vi "FUG-HCN.ProcCases.vi"(0 "i ref in":refnum<vi>, 1 "selector":string, 2 "Data":T1, 3 "call cluster":T2={"Object"="", "Selector"="", "CallType"=enum."synchronous", "Async Object"="", "Async Selector"="", "Data Descriptor"="", "Data"=[], "Error #"=0, "Expire"=0}, 5 "error in (no error)":errorcluster) -> (14 "i ref out":refnum<vi>, 17 "answer cluster":T2={"Object"="", "Selector"="", "CallType"=enum."synchronous", "Async Object"="", "Async Selector"="", "Data Descriptor"="", "Data"=[], "Error #"=0, "Expire"=0}, 19 "error out":errorcluster)   [LabVIEW 2014, in "FUG-HCN.lvlib"]
doc: "This method is called by a process from within the default case in the event loop. The methods of a class that are linked to events will be called from THIS method. Add your code here."
uses:
  FUG-HCN.lvlib
  CS_Core/BaseProcess/BaseProcess.lvlib
  CS_Core/CSSystem/CoreLib/CoreLib.lvlib
  CS_Core/CSSystem/CoreLib/CoreLib.string 2 byte array.vi
  CS_Core/CSSystem/CoreLib/CoreLib.double 2 byte array.vi
  CS_Core/CSSystem/CoreLib/CoreLib.byte array 2 short.vi
  CS_Core/CSSystem/CoreLib/CoreLib.byte array 2 double.vi
  CS_Core/CSSystem/CoreDefs/CoreDefs.call_type.ctl
  CS_Core/BaseProcess/BaseProcess.descriptor string definition.ctl
  CS_Core/CSSystem/CoreDefs/CoreDefs.rawDataType.ctl
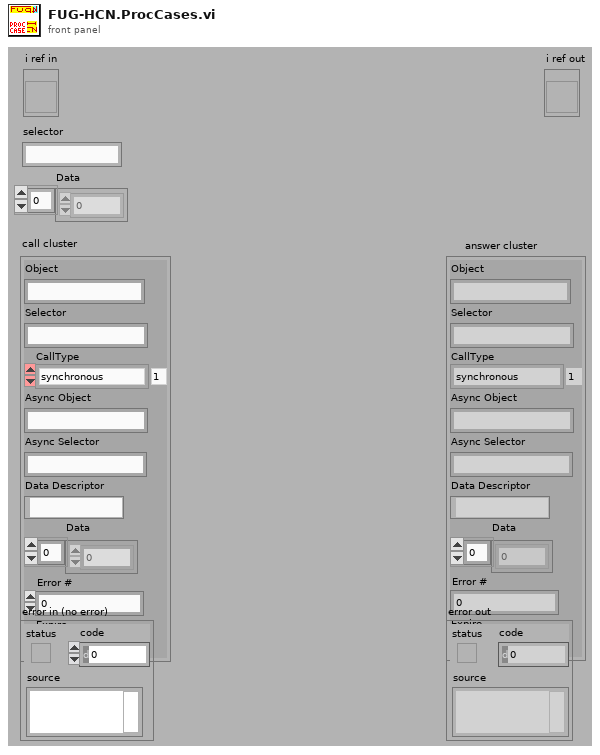
[diagram p1: front panel]
types:
  T1 = typedef "CoreDefs.rawDataType.ctl" = i8[]
  T2 = typedef "CoreDefs.call_type.ctl" = cluster{"Object":string, "Selector":string, "CallType":enum16{"simple", "synchronous", "asynchronous"}, "Async Object":string, "Async Selector":string, "Data Descriptor":T3, "Data":T1, "Error #":i32, "Expire":u32}
  T3 = typedef "BaseProcess.lvlib/BaseProcess.descriptor string definition.ctl" = string
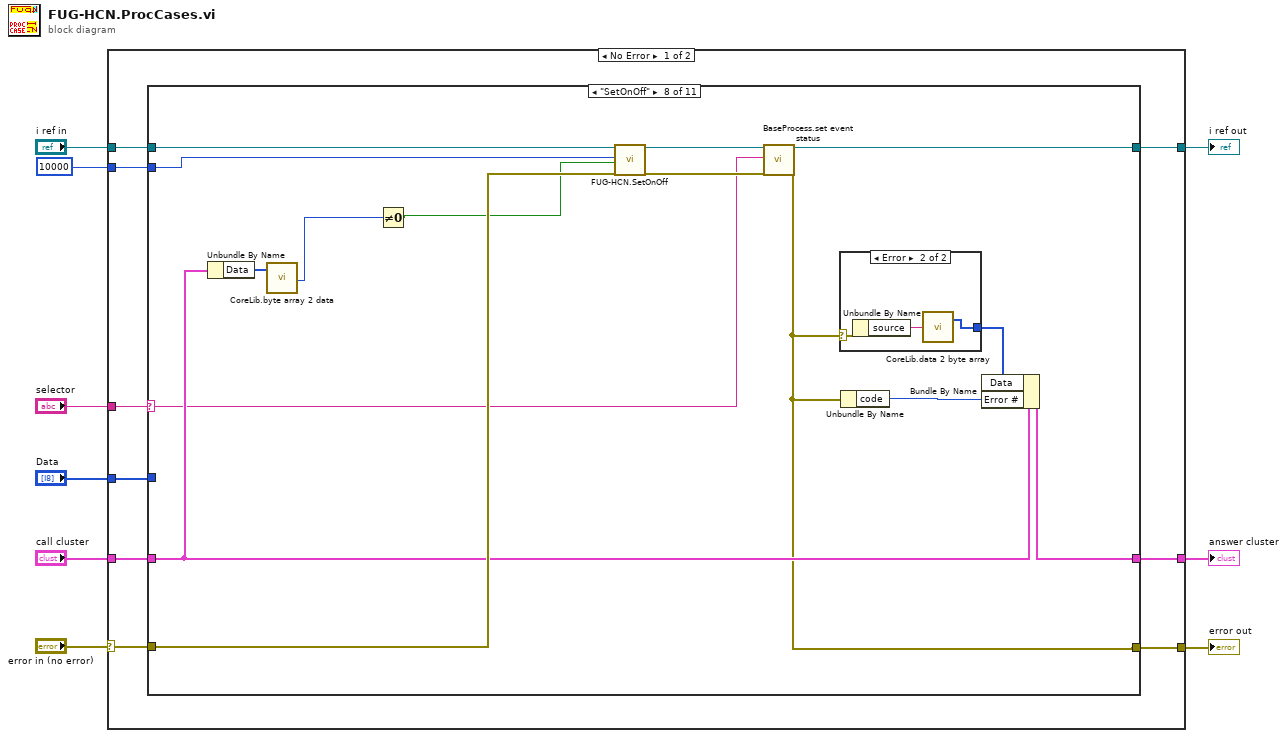
[diagram p0: block diagram]
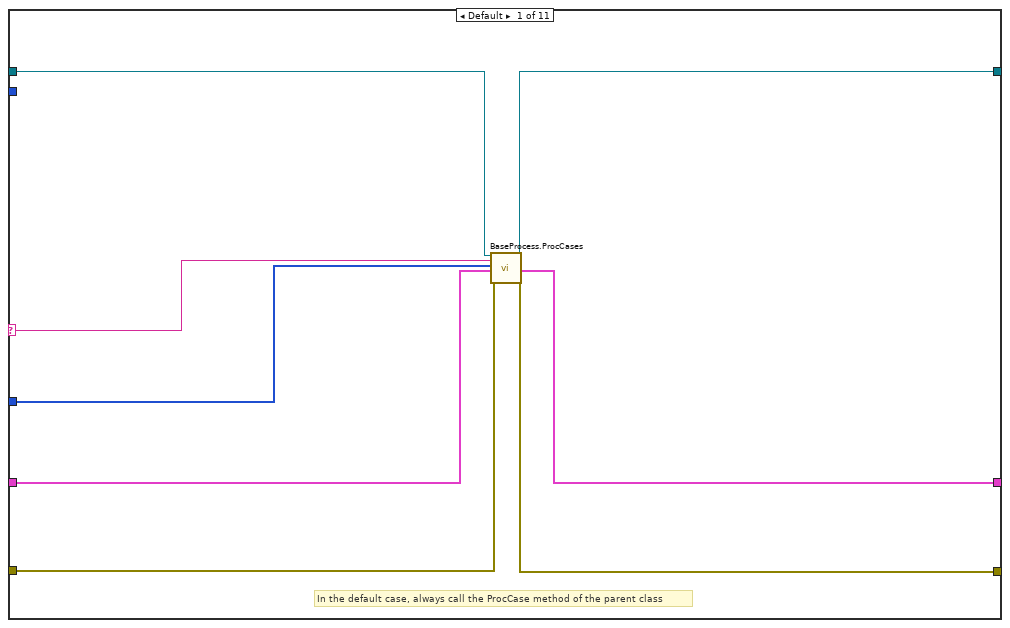
[diagram p2: hidden frame]
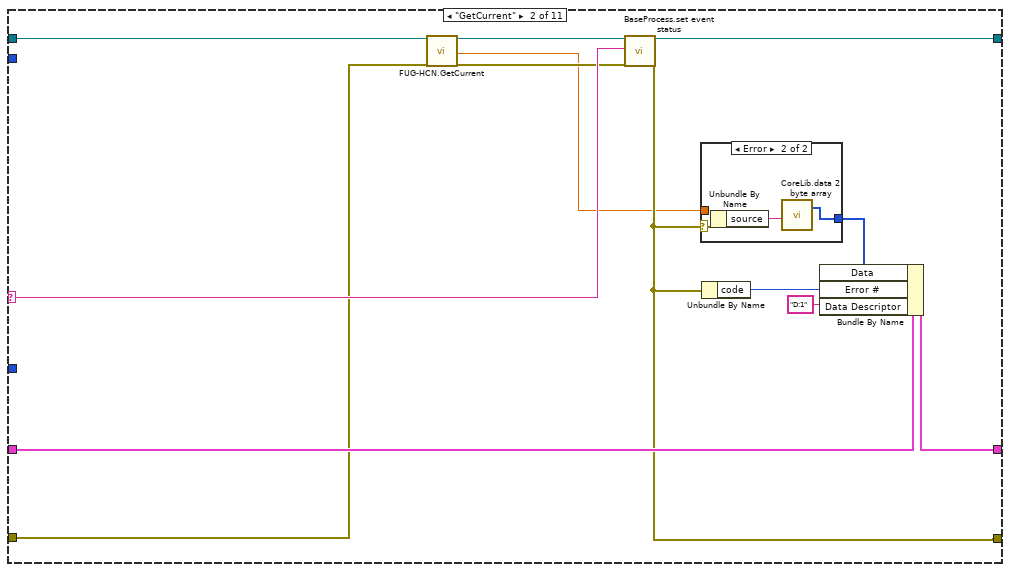
[diagram p3: hidden frame]
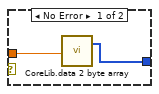
[diagram p4: hidden frame]
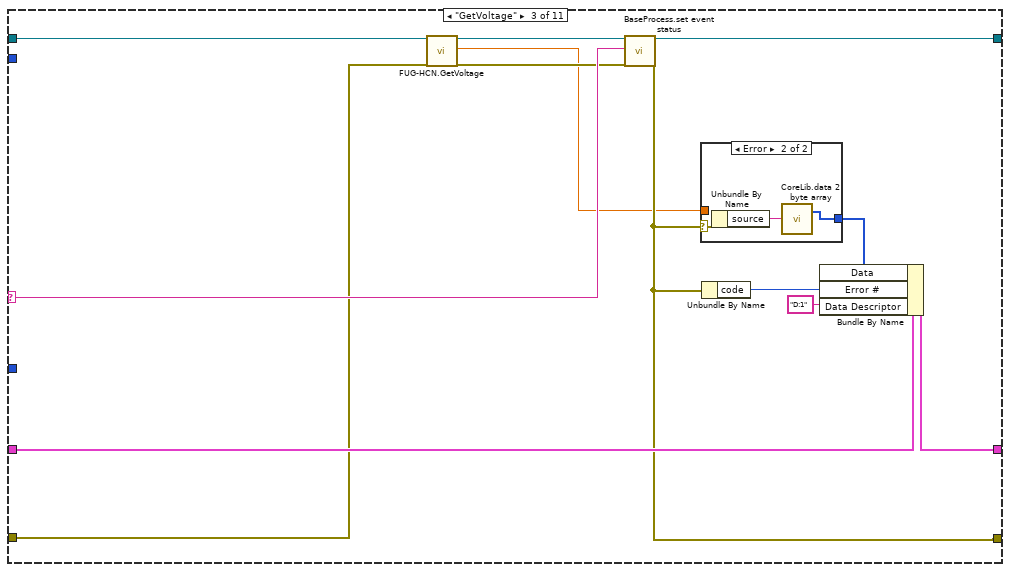
[diagram p5: hidden frame]
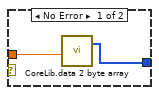
[diagram p6: hidden frame]
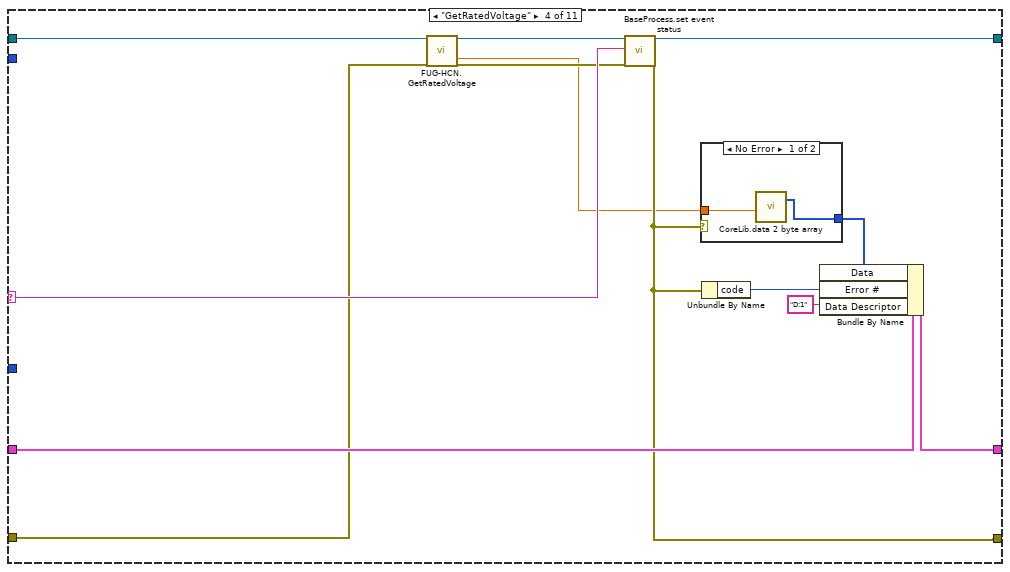
[diagram p7: hidden frame]
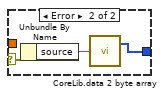
[diagram p8: hidden frame]
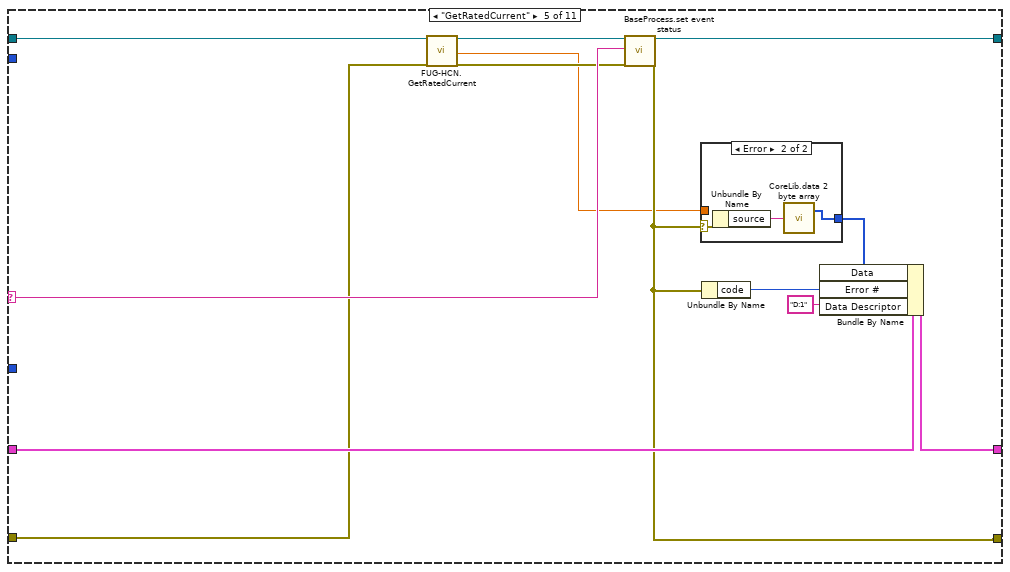
[diagram p9: hidden frame]
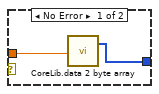
[diagram p10: hidden frame]
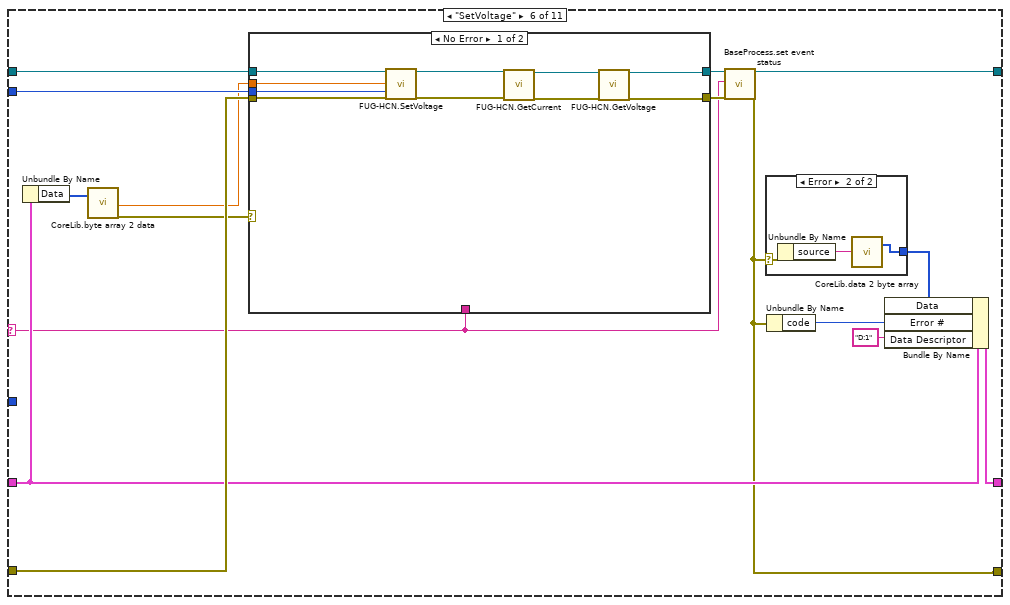
[diagram p11: hidden frame]
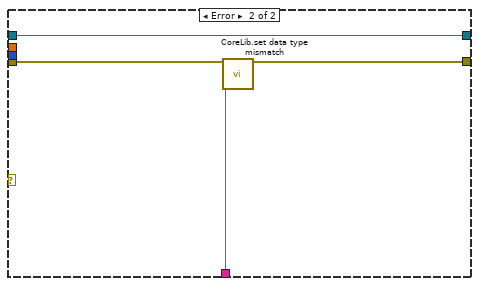
[diagram p13: hidden frame]
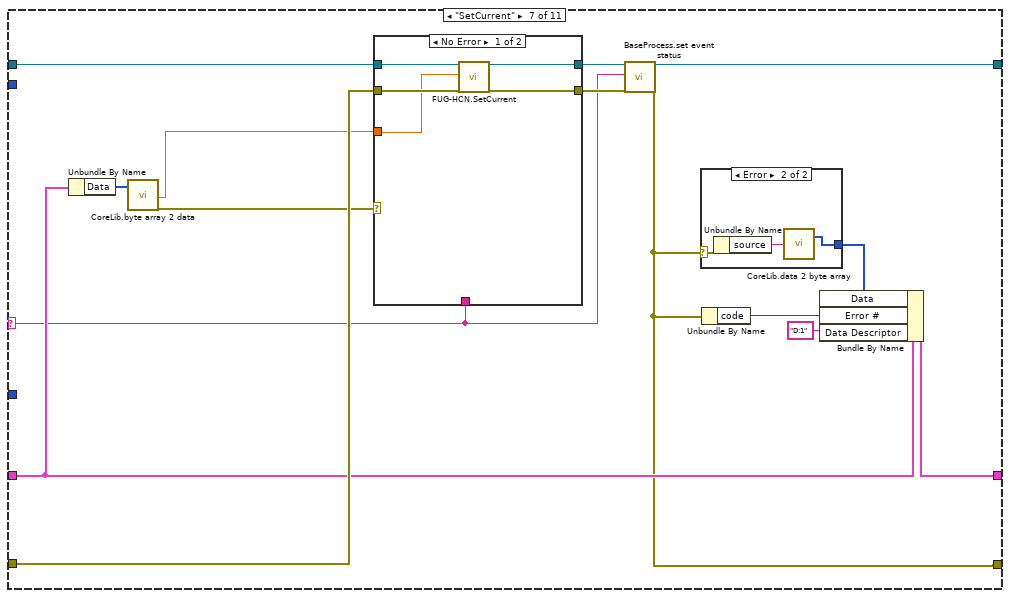
[diagram p14: hidden frame]
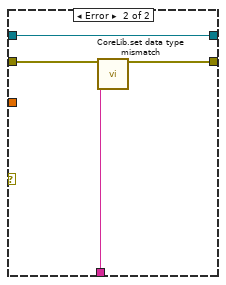
[diagram p16: hidden frame]
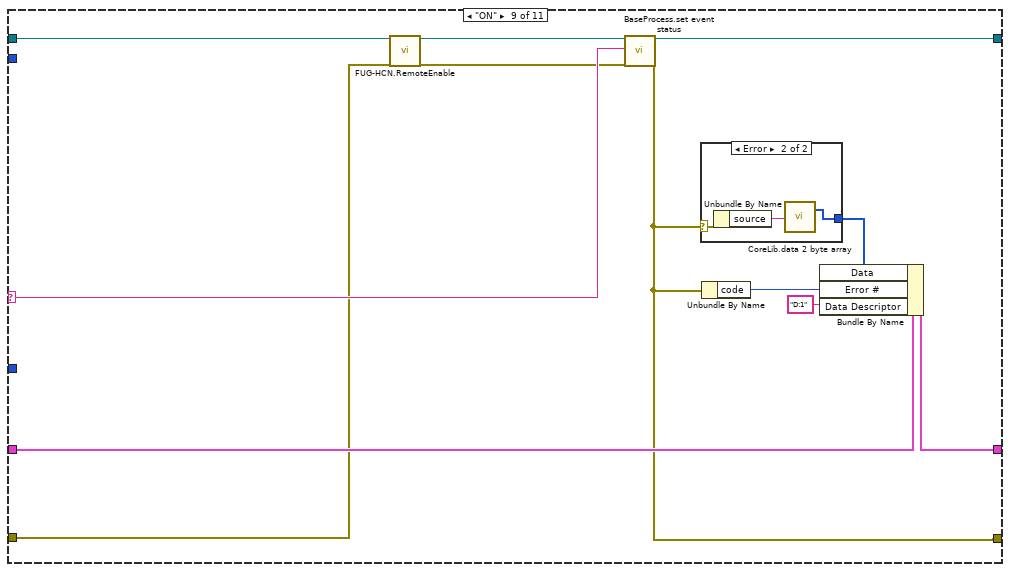
[diagram p18: hidden frame]
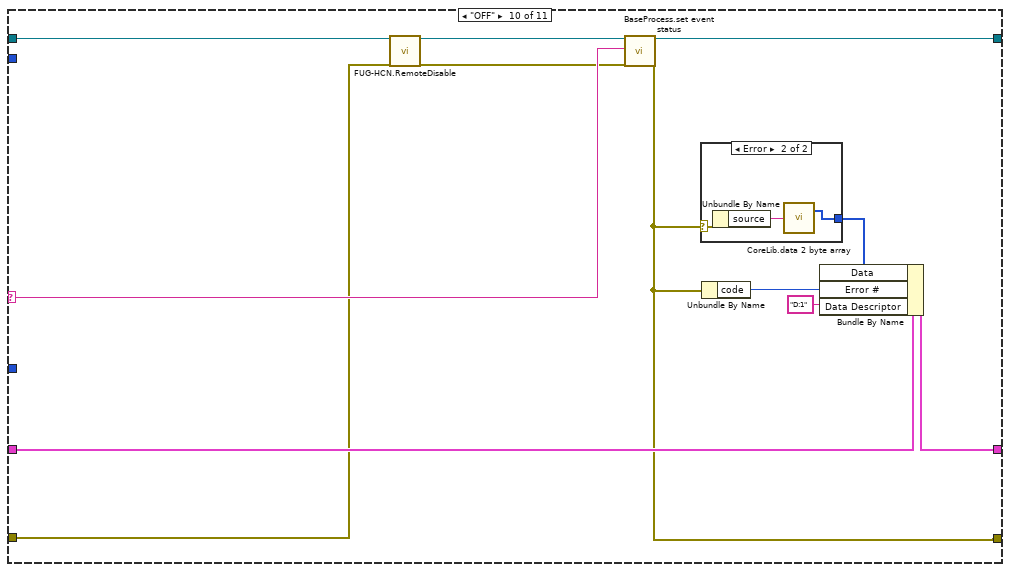
[diagram p20: hidden frame]
diagram:
  n1 = case shown="No Error" "error in (no error)" {
    selector: "error in (no error)" -> [w10 w246]
    tunnel: "selector" -> [w18 _]
    tunnel: [w17 w247] -> w8
    tunnel: "call cluster" -> [w16 w247]
    tunnel: "i ref in" -> [w15 w248]
    tunnel: [w14 w248] -> w5
    tunnel: [w13 w246] -> w4
    tunnel: 10000 -> [w12 _]
    tunnel: "Data" -> [w11 _]
    frame No Error {
      n2 = case shown="\"SetOnOff\"" w18 {
        selector: w18 -> [w20 w34 w52 w70 w88 w105 w137 w164 w183 w198 w214]
        tunnel: w11 -> [w21 _ _ _ _ _ _ _ _ _ _]
        tunnel: w15 -> [w19 w31 w49 w67 w85 w114 w146 w173 w180 w195 w219]
        tunnel: [w26 w33 w51 w69 w87 w104 w136 w163 w182 w197 w221] -> w14
        tunnel: w16 -> [w22 w38 w56 w74 w92 w111 w143 w170 w187 w202 w215]
        tunnel: [w23 w37 w55 w73 w91 w110 w142 w169 w186 w201 w224] -> w17
        tunnel: w10 -> [w25 w29 w47 w65 w83 w113 w145 w172 w178 w193 w217]
        tunnel: [w24 w35 w53 w71 w89 w106 w138 w165 w184 w199 w222] -> w13
        tunnel: w12 -> [_ _ _ _ _ w102 _ w160 _ _ _]
        frame Default {
          # "In the default case, always call the ProcCase method of the parent class"
          n3 = call "BaseProcess.ProcCases.vi"("i ref in"=w19, "selector"=w20, "Data"=w21, "call cluster"=w22, "error in (no error)"=w25) -> ("i ref out"=w26:refnum<vi>, "answer cluster"=w23:T2, "error out"=w24:errorcluster)  [unwired: 12 in]
        }
        frame "GetCurrent" {
          n4 = call "FUG-HCN.GetCurrent.vi"("i ref in"=w31, "error in (no error)"=w29) -> ("i ref out"=w30:refnum<vi>, "Read Current{mA}"=w27:dbl, "error out"=w28:errorcluster)  [unwired: 14 in, 1 out]
          n5 = call "BaseProcess.set event status.vi"("i ref in"=w30, "EventStatus"=w34, "error in (no error)"=w28) -> ("i ref out"=w33:refnum<vi>, "error out"=w35:errorcluster)  [unwired: 14 in, 1 out]
          n6 = case shown="Error" w35 {
            selector: w35 -> [_ w44]
            tunnel: [w40 w42] -> w36
            tunnel: w27 -> [w41 _]
            frame No Error {
              n7 = call-poly "CoreLib.data 2 byte array.vi"("f64"=w41) -> ("byteArray out"=w40:T1)  [unwired: 18 in]
            }
            frame Error {
              n8 = Unbundle By Name(w44) -> ("source"=w43:string)
              n9 = call-poly "CoreLib.data 2 byte array.vi"("string"=w43) -> ("byteArray out"=w42:T1)  [unwired: 18 in]
            }
          }
          n10 = Unbundle By Name(w35) -> ("code"=w39:i32)
          n11 = Bundle By Name(cluster=w38, "Data"=w36, "Error #"=w39, "Data Descriptor"="D:1") -> (w37:T2)
        }
        frame "GetVoltage" {
          n12 = call "FUG-HCN.GetVoltage.vi"("i ref in"=w49, "error in (no error)"=w47) -> ("i ref out"=w48:refnum<vi>, "Read Voltage{V}"=w45:dbl, "error out"=w46:errorcluster)  [unwired: 14 in, 1 out]
          n13 = call "BaseProcess.set event status.vi"("i ref in"=w48, "EventStatus"=w52, "error in (no error)"=w46) -> ("i ref out"=w51:refnum<vi>, "error out"=w53:errorcluster)  [unwired: 14 in, 1 out]
          n14 = case shown="Error" w53 {
            selector: w53 -> [_ w62]
            tunnel: [w58 w60] -> w54
            tunnel: w45 -> [w59 _]
            frame No Error {
              n15 = call-poly "CoreLib.data 2 byte array.vi"("f64"=w59) -> ("byteArray out"=w58:T1)  [unwired: 18 in]
            }
            frame Error {
              n16 = Unbundle By Name(w62) -> ("source"=w61:string)
              n17 = call-poly "CoreLib.data 2 byte array.vi"("string"=w61) -> ("byteArray out"=w60:T1)  [unwired: 18 in]
            }
          }
          n18 = Unbundle By Name(w53) -> ("code"=w57:i32)
          n19 = Bundle By Name(cluster=w56, "Data"=w54, "Error #"=w57, "Data Descriptor"="D:1") -> (w55:T2)
        }
        frame "GetRatedVoltage" {
          n20 = call "FUG-HCN.GetRatedVoltage.vi"("i ref in"=w67, "error in (no error)"=w65) -> ("i ref out"=w66:refnum<vi>, "Rated Voltage{V}"=w63:dbl, "error out"=w64:errorcluster)  [unwired: 14 in, 1 out]
          n21 = call "BaseProcess.set event status.vi"("i ref in"=w66, "EventStatus"=w70, "error in (no error)"=w64) -> ("i ref out"=w69:refnum<vi>, "error out"=w71:errorcluster)  [unwired: 14 in, 1 out]
          n22 = case shown="No Error" w71 {
            selector: w71 -> [_ w80]
            tunnel: [w76 w78] -> w72
            tunnel: w63 -> [w77 _]
            frame No Error {
              n23 = call-poly "CoreLib.data 2 byte array.vi"("f64"=w77) -> ("byteArray out"=w76:T1)  [unwired: 18 in]
            }
            frame Error {
              n24 = Unbundle By Name(w80) -> ("source"=w79:string)
              n25 = call-poly "CoreLib.data 2 byte array.vi"("string"=w79) -> ("byteArray out"=w78:T1)  [unwired: 18 in]
            }
          }
          n26 = Unbundle By Name(w71) -> ("code"=w75:i32)
          n27 = Bundle By Name(cluster=w74, "Data"=w72, "Error #"=w75, "Data Descriptor"="D:1") -> (w73:T2)
        }
        frame "GetRatedCurrent" {
          n28 = call "FUG-HCN.GetRatedCurrent.vi"("i ref in"=w85, "error in (no error)"=w83) -> ("i ref out"=w84:refnum<vi>, "Rated Current{mA}"=w81:dbl, "error out"=w82:errorcluster)  [unwired: 14 in, 1 out]
          n29 = call "BaseProcess.set event status.vi"("i ref in"=w84, "EventStatus"=w88, "error in (no error)"=w82) -> ("i ref out"=w87:refnum<vi>, "error out"=w89:errorcluster)  [unwired: 14 in, 1 out]
          n30 = case shown="Error" w89 {
            selector: w89 -> [_ w98]
            tunnel: [w94 w96] -> w90
            tunnel: w81 -> [w95 _]
            frame No Error {
              n31 = call-poly "CoreLib.data 2 byte array.vi"("f64"=w95) -> ("byteArray out"=w94:T1)  [unwired: 18 in]
            }
            frame Error {
              n32 = Unbundle By Name(w98) -> ("source"=w97:string)
              n33 = call-poly "CoreLib.data 2 byte array.vi"("string"=w97) -> ("byteArray out"=w96:T1)  [unwired: 18 in]
            }
          }
          n34 = Unbundle By Name(w89) -> ("code"=w93:i32)
          n35 = Bundle By Name(cluster=w92, "Data"=w90, "Error #"=w93, "Data Descriptor"="D:1") -> (w91:T2)
        }
        frame "SetVoltage" {
          n36 = Unbundle By Name(w111) -> ("Data"=w101:T1)
          n37 = call-poly "CoreLib.byte array 2 data.vi"("byteArray"=w101) -> ("d64"=w99:dbl, "error out"=w100:errorcluster)  [unwired: 16 in, 1 out]
          n38 = case shown="No Error" w100 {
            tunnel: [w121 w131] -> w108
            tunnel: w114 -> [w126 w131]
            tunnel: w113 -> [w127 w130]
            tunnel: [w122 w129] -> w107
            tunnel: w105 -> [_ w128]
            tunnel: w99 -> [w125 _]
            tunnel: w102 -> [w124 _]
            frame No Error {
              n39 = call "FUG-HCN.SetVoltage.vi"("i ref in"=w126, "Set Voltage"=w125, "Time out"=w124, "error in (no error)"=w127) -> ("i ref out"=w119:refnum<vi>, "error out"=w118:errorcluster)  [unwired: 13 in, 1 out]
              n40 = call "FUG-HCN.GetCurrent.vi"("i ref in"=w119, "error in (no error)"=w118) -> ("i ref out"=w120:refnum<vi>, "error out"=w123:errorcluster)  [unwired: 14 in, 2 out]
              n41 = call "FUG-HCN.GetVoltage.vi"("i ref in"=w120, "error in (no error)"=w123) -> ("i ref out"=w121:refnum<vi>, "error out"=w122:errorcluster)  [unwired: 14 in, 2 out]
            }
            frame Error {
              n42 = call "CoreLib.set data type mismatch.vi"("error in (no error)"=w130, "error source"=w128) -> ("error out"=w129:errorcluster)  [unwired: 17 in]
            }
          }
          n43 = call "BaseProcess.set event status.vi"("i ref in"=w108, "EventStatus"=w105, "error in (no error)"=w107) -> ("i ref out"=w104:refnum<vi>, "error out"=w106:errorcluster)  [unwired: 14 in, 1 out]
          n44 = case shown="Error" w106 {
            selector: w106 -> [_ w117]
            tunnel: [_ w115] -> w109
            frame No Error {
            }
            frame Error {
              n45 = Unbundle By Name(w117) -> ("source"=w116:string)
              n46 = call-poly "CoreLib.data 2 byte array.vi"("string"=w116) -> ("byteArray out"=w115:T1)  [unwired: 18 in]
            }
          }
          n47 = Unbundle By Name(w106) -> ("code"=w112:i32)
          n48 = Bundle By Name(cluster=w111, "Data"=w109, "Error #"=w112, "Data Descriptor"="D:1") -> (w110:T2)
        }
        frame "SetCurrent" {
          n49 = Unbundle By Name(w143) -> ("Data"=w134:T1)
          n50 = call-poly "CoreLib.byte array 2 data.vi"("byteArray"=w134) -> ("d64"=w132:dbl, "error out"=w133:errorcluster)  [unwired: 16 in, 1 out]
          n51 = case shown="No Error" w133 {
            tunnel: [w152 w158] -> w140
            tunnel: w146 -> [w153 w158]
            tunnel: w145 -> [w154 w157]
            tunnel: [w151 w156] -> w139
            tunnel: w137 -> [_ w155]
            tunnel: w132 -> [w150 _]
            frame No Error {
              n52 = call "FUG-HCN.SetCurrent.vi"("i ref in"=w153, "Set Current{mA}"=w150, "error in (no error)"=w154) -> ("i ref out"=w152:refnum<vi>, "error out"=w151:errorcluster)  [unwired: 14 in, 1 out]
            }
            frame Error {
              n53 = call "CoreLib.set data type mismatch.vi"("error in (no error)"=w157, "error source"=w155) -> ("error out"=w156:errorcluster)  [unwired: 17 in]
            }
          }
          n54 = call "BaseProcess.set event status.vi"("i ref in"=w140, "EventStatus"=w137, "error in (no error)"=w139) -> ("i ref out"=w136:refnum<vi>, "error out"=w138:errorcluster)  [unwired: 14 in, 1 out]
          n55 = case shown="Error" w138 {
            selector: w138 -> [_ w149]
            tunnel: [_ w147] -> w141
            frame No Error {
            }
            frame Error {
              n56 = Unbundle By Name(w149) -> ("source"=w148:string)
              n57 = call-poly "CoreLib.data 2 byte array.vi"("string"=w148) -> ("byteArray out"=w147:T1)  [unwired: 18 in]
            }
          }
          n58 = Unbundle By Name(w138) -> ("code"=w144:i32)
          n59 = Bundle By Name(cluster=w143, "Data"=w141, "Error #"=w144, "Data Descriptor"="D:1") -> (w142:T2)
        }
        frame "SetOnOff" {
          n60 = Unbundle By Name(w170) -> ("Data"=w162:T1)
          n61 = call-poly "CoreLib.byte array 2 data.vi"("byteArray"=w162) -> ("i16"=w161:i16)  [unwired: 16 in, 2 out]
          n62 = Not Equal To 0?(x=w161) -> (x != 0?=w159:bool)
          n63 = call "FUG-HCN.SetOnOff.vi"("i ref in"=w173, "Time out"=w160, "on (FALSE)"=w159, "error in (no error)"=w172) -> ("i ref out"=w167:refnum<vi>, "error out"=w166:errorcluster)  [unwired: 14 in]
          n64 = call "BaseProcess.set event status.vi"("i ref in"=w167, "EventStatus"=w164, "error in (no error)"=w166) -> ("i ref out"=w163:refnum<vi>, "error out"=w165:errorcluster)  [unwired: 14 in, 1 out]
          n65 = case shown="Error" w165 {
            selector: w165 -> [_ w176]
            tunnel: [_ w174] -> w168
            frame No Error {
            }
            frame Error {
              n66 = Unbundle By Name(w176) -> ("source"=w175:string)
              n67 = call-poly "CoreLib.data 2 byte array.vi"("string"=w175) -> ("byteArray out"=w174:T1)  [unwired: 18 in]
            }
          }
          n68 = Unbundle By Name(w165) -> ("code"=w171:i32)
          n69 = Bundle By Name(cluster=w170, "Data"=w168, "Error #"=w171) -> (w169:T2)
        }
        frame "ON" {
          n70 = call "FUG-HCN.RemoteEnable.vi"("i ref in"=w180, "error in (no error)"=w178) -> ("i ref out"=w179:refnum<vi>, "error out"=w177:errorcluster)  [unwired: 15 in, 1 out]
          n71 = call "BaseProcess.set event status.vi"("i ref in"=w179, "EventStatus"=w183, "error in (no error)"=w177) -> ("i ref out"=w182:refnum<vi>, "error out"=w184:errorcluster)  [unwired: 14 in, 1 out]
          n72 = case shown="Error" w184 {
            selector: w184 -> [_ w191]
            tunnel: [_ w189] -> w185
            frame No Error {
            }
            frame Error {
              n73 = Unbundle By Name(w191) -> ("source"=w190:string)
              n74 = call-poly "CoreLib.data 2 byte array.vi"("string"=w190) -> ("byteArray out"=w189:T1)  [unwired: 18 in]
            }
          }
          n75 = Unbundle By Name(w184) -> ("code"=w188:i32)
          n76 = Bundle By Name(cluster=w187, "Data"=w185, "Error #"=w188, "Data Descriptor"="D:1") -> (w186:T2)
        }
        frame "OFF" {
          n77 = call "FUG-HCN.RemoteDisable.vi"("i ref in"=w195, "error in (no error)"=w193) -> ("i ref out"=w194:refnum<vi>, "error out"=w192:errorcluster)  [unwired: 15 in, 1 out]
          n78 = call "BaseProcess.set event status.vi"("i ref in"=w194, "EventStatus"=w198, "error in (no error)"=w192) -> ("i ref out"=w197:refnum<vi>, "error out"=w199:errorcluster)  [unwired: 14 in, 1 out]
          n79 = case shown="Error" w199 {
            selector: w199 -> [_ w206]
            tunnel: [_ w204] -> w200
            frame No Error {
            }
            frame Error {
              n80 = Unbundle By Name(w206) -> ("source"=w205:string)
              n81 = call-poly "CoreLib.data 2 byte array.vi"("string"=w205) -> ("byteArray out"=w204:T1)  [unwired: 18 in]
            }
          }
          n82 = Unbundle By Name(w199) -> ("code"=w203:i32)
          n83 = Bundle By Name(cluster=w202, "Data"=w200, "Error #"=w203, "Data Descriptor"="D:1") -> (w201:T2)
        }
        frame "Remote" {
          n84 = Unbundle By Name(w215) -> ("Data"=w210:T1)
          n85 = call-poly "CoreLib.byte array 2 data.vi"("byteArray"=w210) -> ("i16"=w208:i16, "error out"=w209:errorcluster)  [unwired: 16 in, 1 out]
          n86 = Equal To 0?(x=w208) -> (x = 0?=w211:bool)
          n87 = Select(t=FALSE, s=w211, f=TRUE) -> (s? t:f=w207:bool)
          n88 = case shown="No Error" w209 {
            tunnel: w219 -> [w230 w239]
            tunnel: [w229 w239] -> w218
            tunnel: w217 -> [w228 w242]
            tunnel: [w227 w241] -> w216
            tunnel: w207 -> [w226 _]
            tunnel: w214 -> [_ w240]
            frame No Error {
              n89 = case shown="False" w226 {
                tunnel: w230 -> [w234 w238]
                tunnel: [w233 w237] -> w229
                tunnel: w228 -> [w232 w235]
                tunnel: [w231 w236] -> w227
                frame False {
                  n90 = call "FUG-HCN.RemoteDisable.vi"("i ref in"=w234, "error in (no error)"=w232) -> ("i ref out"=w233:refnum<vi>, "error out"=w231:errorcluster)  [unwired: 15 in, 1 out]
                }
                frame True {
                  n91 = call "FUG-HCN.RemoteEnable.vi"("i ref in"=w238, "error in (no error)"=w235) -> ("i ref out"=w237:refnum<vi>, "error out"=w236:errorcluster)  [unwired: 15 in, 1 out]
                }
              }
            }
            frame Error {
              n92 = call "CoreLib.set data type mismatch.vi"("error in (no error)"=w242, "error source"=w240) -> ("error out"=w241:errorcluster)  [unwired: 17 in]
            }
          }
          n93 = call "BaseProcess.set event status.vi"("i ref in"=w218, "EventStatus"=w214, "error in (no error)"=w216) -> ("i ref out"=w221:refnum<vi>, "error out"=w222:errorcluster)  [unwired: 14 in, 1 out]
          n94 = case shown="Error" w222 {
            selector: w222 -> [_ w245]
            tunnel: [_ w243] -> w223
            frame No Error {
            }
            frame Error {
              n95 = Unbundle By Name(w245) -> ("source"=w244:string)
              n96 = call-poly "CoreLib.data 2 byte array.vi"("string"=w244) -> ("byteArray out"=w243:T1)  [unwired: 18 in]
            }
          }
          n97 = Unbundle By Name(w222) -> ("code"=w225:i32)
          n98 = Bundle By Name(cluster=w215, "Data"=w223, "Error #"=w225, "Data Descriptor"="D:1") -> (w224:T2)
        }
      }
    }
    frame Error {
    }
  }
  "answer cluster" <- w8
  "i ref out" <- w5
  "error out" <- w4
